vi "Sub_Build_MQTT_String.vi"(8 "error in (no error)":errorcluster, 10 "String to be encoded":string="MQIsdp") -> (0 "error out":errorcluster, 2 "UTF8 Byte Array":u8[](array[numeric]) format="%x")   [LabVIEW 2019, in "MQTT_Functions.lvlib"]
uses:
  MQTT_Functions.lvlib
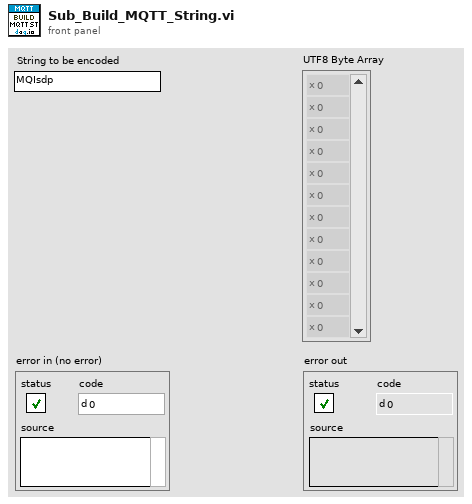
[diagram p1: front panel]
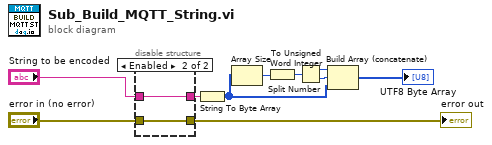
[diagram p0: block diagram]
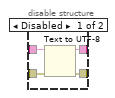
[diagram p2: hidden frame]
diagram:
  n1 = disable-structure shown="Enabled" {
    disable-tunnel: "String to be encoded" -> [w14 w16]
    disable-tunnel: "error in (no error)" -> [w13 w15]
    disable-tunnel: [w12 w16] -> w8
    disable-tunnel: [w11 w15] -> w1
    frame Disabled {
      n2 = Text to UTF-8(8:w13, 11:w14) -> (0:w11:errorcluster, 3:w12:string)  [unwired: 1 in]
    }
    frame Enabled {
    }
  }
  "error out" <- w1
  n3 = String To Byte Array(string=w8) -> (unsigned byte array=w7:u8[])
  n4 = Array Size(array=w7) -> (size(s)=w6:i32)
  n5 = To Unsigned Word Integer(number=w6) -> (unsigned 16bit integer=w2:u16)
  n6 = Split Number(x=w2) -> (hi(x)=w4:u8, lo(x)=w5:u8)
  n7 = Build Array (concatenate)(w4, w5, w7) -> (→"UTF8 Byte Array":u8[])
